vi "SetJogStep_KCubeInertial.vi"(9 "JogStepFwd in":i32=500, 10 "JogStepRev in":i32=250, 11 ".NET Refnum in":refnum<k24>) -> (2 "JogStepFwd out":i32, 3 "JogStepRev out":i32)   [LabVIEW 2019]
doc: "set and get relative position values for inertial motor"
uses:
  D:/Victor Sun/optical trap control/Kinesis/Thorlabs.MotionControl.KCube.InertialMotorCLI.dll
  Kinesis/Thorlabs.MotionControl.KCube.InertialMotorCLI.dll
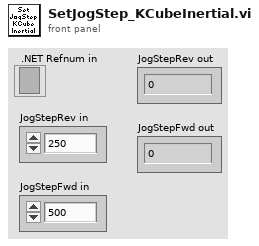
[diagram p1: front panel]
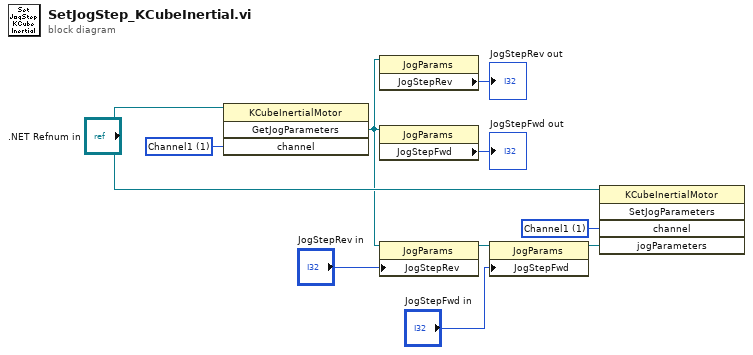
[diagram p0: block diagram]
diagram:
  w8 = 1 items=["Channel1"=1, "Channel2"=2, "Channel3"=3, "Channel4"=4] ("channel")
  w3 = 1 items=["Channel1"=1, "Channel2"=2, "Channel3"=3, "Channel4"=4] ("channel")
  n1 = invoke class="KCubeInertialMotor" method="GetJogParameters"(reference=".NET Refnum in", "channel"=w3) -> ("GetJogParameters"=w6:refnum<k24>)  [unwired: 2 in, 3 out]
  n2 = property class="JogParams"(reference=w6) -> ("JogStepRev"=→"JogStepRev out":i32)  [unwired: 1 in, 2 out]
  n3 = property class="JogParams"(reference=w6) -> ("JogStepFwd"=→"JogStepFwd out":i32)  [unwired: 1 in, 2 out]
  n4 = property class="JogParams"(reference=w6, "JogStepRev"="JogStepRev in") -> (reference out=w7:refnum<k24>)  [unwired: 1 in, 1 out]
  n5 = property class="JogParams"(reference=w7, "JogStepFwd"="JogStepFwd in") -> (reference out=w9:refnum<k24>)  [unwired: 1 in, 1 out]
  n6 = invoke class="KCubeInertialMotor" method="SetJogParameters"(reference=".NET Refnum in", "channel"=w8, "jogParameters"=w9) -> ()  [unwired: 2 in, 5 out]
